vi "Init.vi"(8 "Path":path, 9 "Register":refnum<event-registration>, 10 "Addresses Strategy":refnum<class "Addresses Strategy.lvclass">) -> (3 "Base Actor out":refnum<class "Base Actor.lvclass">)   [LabVIEW 2021, in "jettl.lvlib" / "Actor.lvlib" / "Base Actor.lvclass"]
uses:
  Base Actor.lvclass
  Addresses Strategy/Addresses Strategy/Addresses Strategy.lvclass
  Msg/Msg.lvclass
  Base Actor.lvclass/Base Actor.ctl
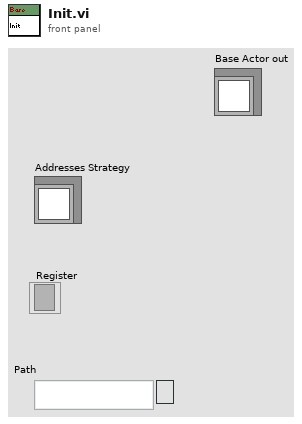
[diagram p1: front panel]
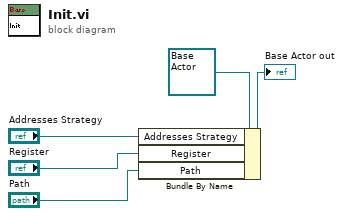
[diagram p0: block diagram]
diagram:
  n1 = Bundle By Name(cluster=refnum<class "Base Actor.lvclass"> refnum ("jettl Event Actor out"), "Addresses Strategy"="Addresses Strategy", "Register"="Register", "Path"="Path") -> (→"Base Actor out":refnum<class "Base Actor.lvclass">)
